vi "MovePossible_MoveComplete.vi"(1 "Axis Array":string[](array[string]), 2 "Position Array":dbl[](array[numeric]), 3 "error in (no error)":errorcluster) -> (8 "Axis moving?":bool[](array[boolean]), 9 "Move possible":bool, 10 "error out":errorcluster)   [LabVIEW 2020]
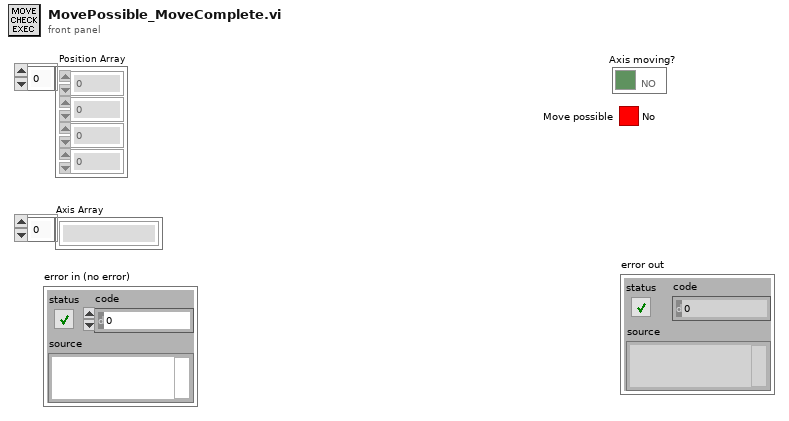
[diagram p1: front panel]
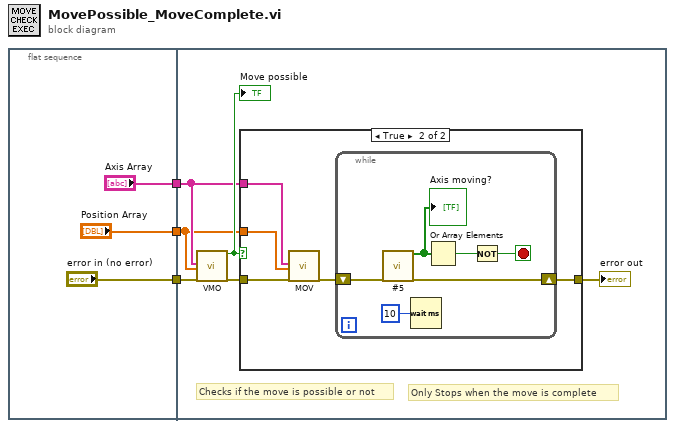
[diagram p0: block diagram]
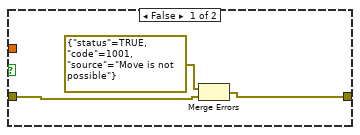
[diagram p2: hidden frame]
diagram:
  n1 = flat-sequence {
    tunnel: ["error in (no error)"] -> w3
    tunnel: ["Position Array"] -> w2
    tunnel: ["Axis Array"] -> w1
    tunnel: w3 -> [w9]
    tunnel: w2 -> [w7]
    tunnel: w1 -> [w8]
    frame #0 {
    }
    frame #1 {
      # "Checks if the move is possible or not"
      # "Only Stops when the move is complete"
      n2 = call "VMO.vi"("Axes to command"=w8, "Position values"=w7, "error in"=w9) -> ("Move possible"=w12:bool, "error out"=w11:errorcluster)  [unwired: 15 in]
      "Move possible" <- w12
      n3 = case shown="True" w12 {
        tunnel: [w14 w20] -> w10
        tunnel: w11 -> [w15 w19]
        tunnel: w8 -> [_ w17]
        tunnel: w7 -> [_ w16]
        frame False {
          n4 = Merge Errors(errorcluster {"status"=TRUE, "code"=1001, "source"="Move is not possible"} ("error in"), w15) -> (w14:errorcluster)
        }
        frame True {
          n5 = call "MOV.vi"("Axes to move"=w17, "Position values"=w16, "error in"=w19) -> ("error out"=w18:errorcluster)  [unwired: 16 in]
          n6 = while {
            shift-right: [w25] -> w20
            shift-left: w18 -> [w26]
            stop <- w21 stop-if-true
            n7 = call "#5.vi"("error in"=w26) -> ("Axis moving?"=w23:bool[], "error out"=w25:errorcluster)  [unwired: 17 in]
            "Axis moving?" <- w23
            n8 = Wait (ms)(milliseconds to wait=u32 10) -> ()  [unwired: 1 out]
            n9 = Or Array Elements(Boolean array=w23) -> (logical OR=w22:bool)
            n10 = Not(x=w22) -> (.not. x?=w21:bool)
          }
        }
      }
      "error out" <- w10
    }
  }
